vi "Get Digest.vi"(11 "Hash Function in":refnum<class "NI_SHA-256.lvclass">) -> (2 "Digest":u8[](array[numeric]) format="%02x", 3 "Hash Function out":refnum<class "NI_SHA-256.lvclass">)   [LabVIEW 2020, in "NI_SHA-256.lvclass"]
doc: "Compute the message digest given previously supplied input blocks."
uses:
  <vilib>/security/Message Digest/SHA-2/SHA-256/NI_SHA-256.lvclass
  <vilib>/security/Message Digest/SHA-2/SHA-256/NI_SHA-256.lvclass/NI_SHA-256.ctl
  <vilib>/Bit Manipulation/wrappers/Words To Network-Order Bytes/Words To Network-Order Bytes U32.vi
  <vilib>/Bit Manipulation/NI_Bit Manipulation.lvlib
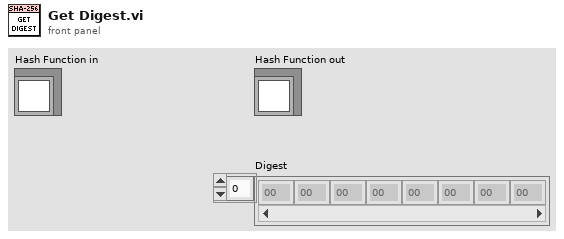
[diagram p1: front panel]
types:
  T1 = typedef "NI_SHA-256.lvclass/Mode.ctl" = enum16{"SHA-256", "SHA-224"}
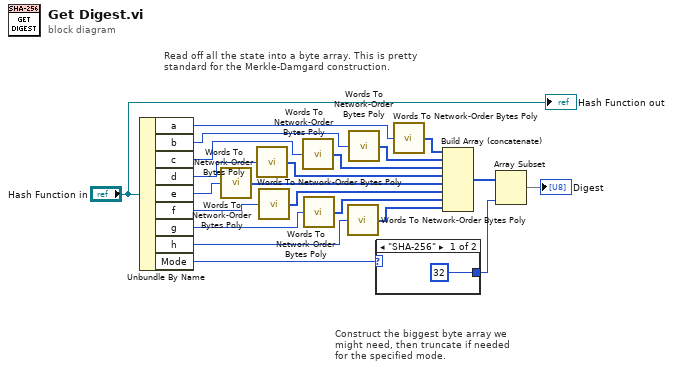
[diagram p0: block diagram]
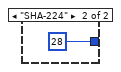
[diagram p2: hidden frame]
diagram:
  # "Construct the biggest byte array we might need, then truncate if needed for the specified mode."
  # "Read off all the state into a byte array. This is pretty standard for the Merkle-Damgard construction."
  n1 = Unbundle By Name("Hash Function in") -> ("a"=w21:u32, "b"=w14:u32, "c"=w13:u32, "d"=w12:u32, "e"=w11:u32, "f"=w10:u32, "g"=w9:u32, "h"=w8:u32, "Mode"=w17:T1)
  n2 = call-poly <vilib>:"Words To Network-Order Bytes Poly.vi"("word"=w11) -> ("bytes"=w4:u8[])
  n3 = call-poly <vilib>:"Words To Network-Order Bytes Poly.vi"("word"=w12) -> ("bytes"=w3:u8[])
  n4 = call-poly <vilib>:"Words To Network-Order Bytes Poly.vi"("word"=w10) -> ("bytes"=w5:u8[])
  n5 = call-poly <vilib>:"Words To Network-Order Bytes Poly.vi"("word"=w13) -> ("bytes"=w2:u8[])
  n6 = call-poly <vilib>:"Words To Network-Order Bytes Poly.vi"("word"=w9) -> ("bytes"=w6:u8[])
  n7 = call-poly <vilib>:"Words To Network-Order Bytes Poly.vi"("word"=w8) -> ("bytes"=w7:u8[])
  n8 = call-poly <vilib>:"Words To Network-Order Bytes Poly.vi"("word"=w14) -> ("bytes"=w1:u8[])
  n9 = case shown="\"SHA-256\"" w17 {
    tunnel: [32 28] -> w16
    frame "SHA-256" {
    }
    frame "SHA-224" {
    }
  }
  n10 = call-poly <vilib>:"Words To Network-Order Bytes Poly.vi"("word"=w21) -> ("bytes"=w19:u8[])
  n11 = Build Array (concatenate)(w19, w1, w2, w3, w4, w5, w6, w7) -> (w18:u8[])
  n12 = Array Subset(array=w18, length=w16) -> (→"Digest":u8[])  [unwired: 1 in]
  "Hash Function out" <- "Hash Function in"
